vi "单用户自定义事件界面程序.vi"() -> ()   [LabVIEW 2009]
doc: "本VI是为《我和LabVIEW》一书编写的示例。\n关于本书的介绍请参考网页：\nhttp://ruanqizhen.spaces.live.com/blog/cns!5852D4F797C53FB6!4310.entry"
uses:
  C:/Program Files/National Instruments/LabVIEW 2009/resource/importtools/Common/Event/NISAST Event.lvclass
panel:
  in  "停止":bool
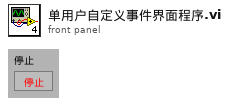
[diagram p1: front panel]
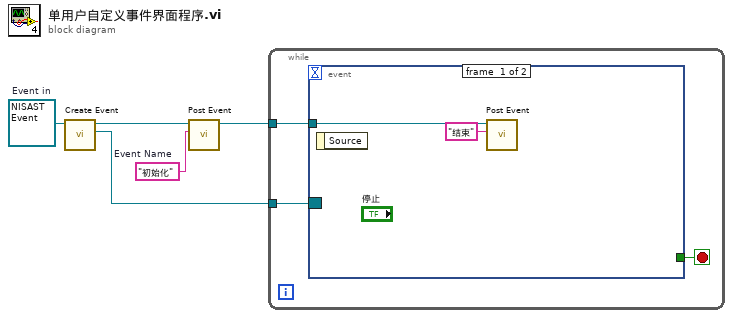
[diagram p0: block diagram]
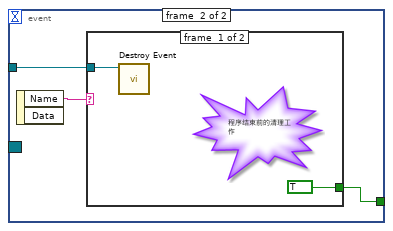
[diagram p2: hidden frame]
diagram:
  w1 = "初始化"  # Event Name
  w4 = refnum<class "NISAST Event.lvclass"> refnum  # Event in
  n1 = call-dynamic "Create Event.vi"("Event in"=w4) -> ("Event Registration Refnum"=w5:refnum<event-registration>, "Event out"=w3:refnum<class "NISAST Event.lvclass">)  [unwired: 1 in, 8 out]
  n2 = call-dynamic "Post Event.vi"("Event Name"=w1, "Event in"=w3) -> ("Event out"=w2:refnum<class "NISAST Event.lvclass">)  [unwired: 2 in, 7 out]
  n3 = while {
    tunnel: w5 -> [w8]
    tunnel: w2 -> [w6]
    stop <- w7 stop-if-true
    n4 = event shown="[1] <User Event>: User Event" {
      selector: w8 -> [_ _]
      dyn-events: _ -> [_ _]
      timeout: _ -> [_ _]
      tunnel: [_ w12] -> w7
      tunnel: w6 -> [w10 w11]
      event #0 {
        n5 = event-data() -> ()  [unwired: 2 out]
        n6 = call-dynamic "Post Event.vi"("Event Name"="结束", "Event in"=w10) -> ()  [unwired: 2 in, 8 out]
      }
      event #1 {
        n7 = event-data() -> ("Name"=w13:string)  [unwired: 2 out]
        n8 = case shown="\"初始化\", Default" w13 {
          tunnel: [TRUE ("停止") _] -> w12
          tunnel: w11 -> [w14 _]
          frame #0 {
            # "程序结束前的清理工作"
            n9 = call-dynamic "Destroy Event.vi"("Event in"=w14) -> ()  [unwired: 1 in, 10 out]
          }
          frame #1 {
            # "程序初始化工作"
          }
        }
      }
    }
  }
